vi "SerialString_to_Ints.vi"(3 "input string":string) -> (18 "output 9":i32, 19 "output 10":i32, 20 "output 1":i32, 21 "output 2":i32, 22 "output 3":i32, 23 "output 4":i32, 24 "output 5":i32, 25 "output 6":i32, 26 "output 7":i32, 27 "output 8":i32)   [LabVIEW 2020]
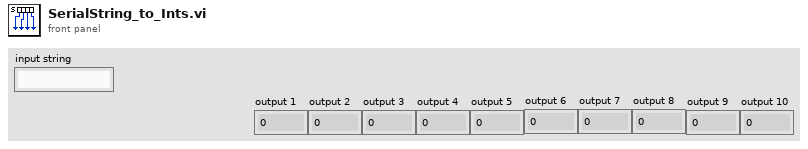
[diagram p1: front panel]
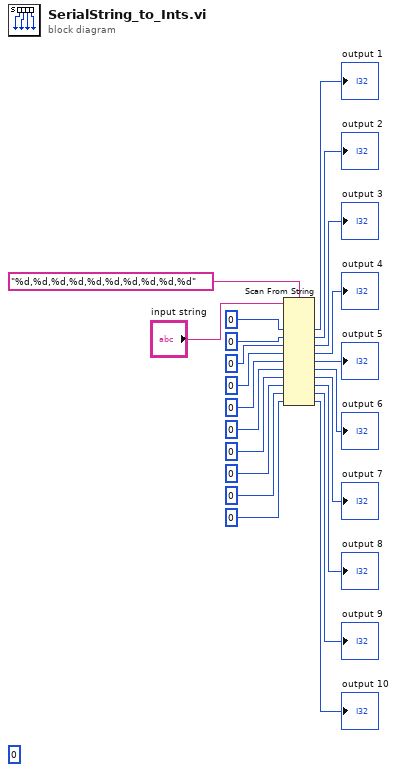
[diagram p0: block diagram]
diagram:
  (unwired) 0 ("default value 2")
  n1 = Scan From String(format string="%d,%d,%d,%d,%d,%d,%d,%d,%d,%d", input string="input string", default 1=0 ("default value 1"), default 2=0 ("default value 2"), default 3=0 ("default value 3"), default 4=0 ("default value 4"), default 5=0 ("default value 5"), default 6=0 ("default value 6"), default 7=0 ("default value 7"), default 8=0 ("default value 8"), default 9=0 ("default value 9"), default 10=0 ("default value 10")) -> (output 1=→"output 1":i32, output 2=→"output 2":i32, output 3=→"output 3":i32, output 4=→"output 4":i32, output 5=→"output 5":i32, output 6=→"output 6":i32, output 7=→"output 7":i32, output 8=→"output 8":i32, output 9=→"output 9":i32, output 10=→"output 10":i32)  [unwired: 2 in, 3 out]
